vi "File.Delete File if Exists.vi"(8 "error in":errorcluster, 11 "Path":path) -> (0 "error out":errorcluster, 3 "Path Out":path)   [LabVIEW 2024]
uses:
  File Utils.lvlib
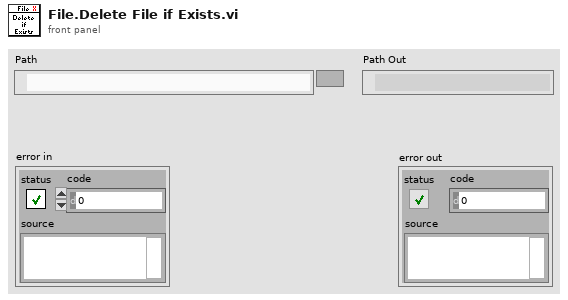
[diagram p1: front panel]
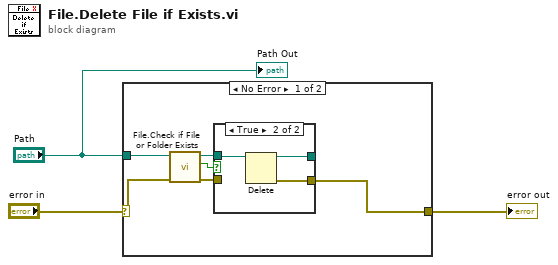
[diagram p0: block diagram]
diagram:
  n1 = case shown="No Error" "error in" {
    selector: "error in" -> [w5 w14]
    tunnel: "Path" -> [w7 _]
    tunnel: [w4 w14] -> w2
    frame No Error {
      n2 = call "File.Check if File or Folder Exists.vi"("error in"=w5, "Path"=w7) -> ("error out"=w6:errorcluster, "Exists"=w9:bool, "Dup Path"=w8:path)  [unwired: 5 in, 2 out]
      n3 = case shown="True" w9 {
        tunnel: w8 -> [w10 w13]
        tunnel: [_ w12] -> w4
        tunnel: [w10 w11] -> _
        tunnel: w6 -> [_ _]
        frame False {
        }
        frame True {
          n4 = Delete(path (use dialog)=w13) -> (deleted path=w11:path, error out=w12:errorcluster)  [unwired: 4 in, 1 out]
        }
      }
    }
    frame Error {
    }
  }
  "error out" <- w2
  "Path Out" <- "Path"
